vi "Create.vi"(8 "error in (no error)":errorcluster, 9 "Startup Promise":refnum<class "Promise.lvclass">, 10 "App":refnum<class "App.lvclass">) -> (0 "error out":errorcluster, 3 "VolatusCore out":refnum<class "VolatusCore.lvclass">)   [LabVIEW 2020, in "Volatus.lvlib" / "VolatusCore.lvclass"]
uses:
  VolatusCore.lvclass
  VolatusCore.lvclass/VolatusCore.ctl
  App/App.lvclass
  lv-promises/Promises/Promise/Promise.lvclass
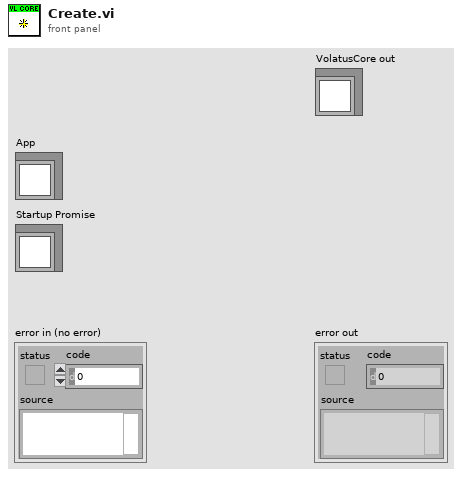
[diagram p1: front panel]
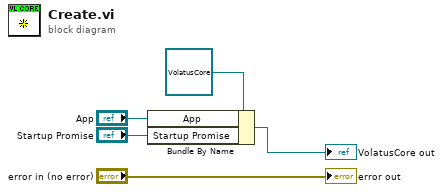
[diagram p0: block diagram]
diagram:
  n1 = Bundle By Name(cluster=refnum<class "VolatusCore.lvclass"> refnum ("VolatusCore in"), "App"="App", "Startup Promise"="Startup Promise") -> (→"VolatusCore out":refnum<class "VolatusCore.lvclass">)
  "error out" <- "error in (no error)"
